vi "Singleton.vi"(8 "error in (no error)":errorcluster) -> (0 "error out":errorcluster, 1 "RequestQueue":refnum<queue>, 3 "MDPtrMgrDVR":refnum<data-value>)   [LabVIEW 2017, in "MDPtr.lvlib" / "MDPtrMgr.lvclass"]
uses:
  MDPtrMgr.lvclass
  Factory/Def-Request.ctl
  Factory/Def-Respone.ctl
  MDPtr TypeDef/MDPtr DataFrame-Memory.ctl
  MDPtr TypeDef/MDPtr DataFrame-Common.ctl
  <vilib>/Utility/Data Type/Type Definitions/Data Type.ctl
  Factory/Def-MDPtrQ.ctl
  <vilib>/Utility/Data Type/NI_Data Type.lvlib
  MDPtr.lvlib
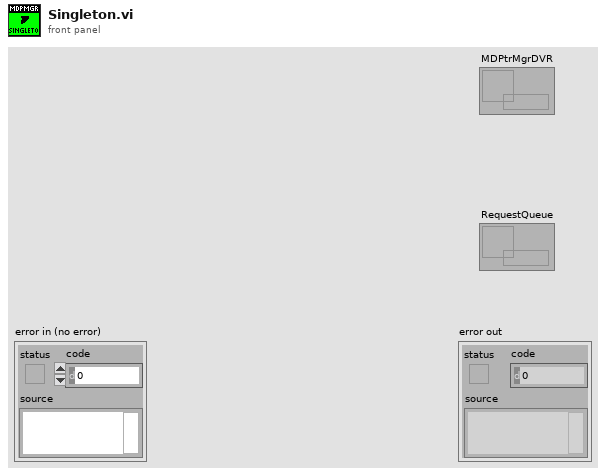
[diagram p1: front panel]
types:
  T1 = typedef "MDPtr.lvlib/MDPtrMgr.lvclass/Def-Request.ctl" = cluster{"Type":enum16{"DVR", "Queue"}, "Cache Length":i32, "ResponeQueue":refnum<queue>}
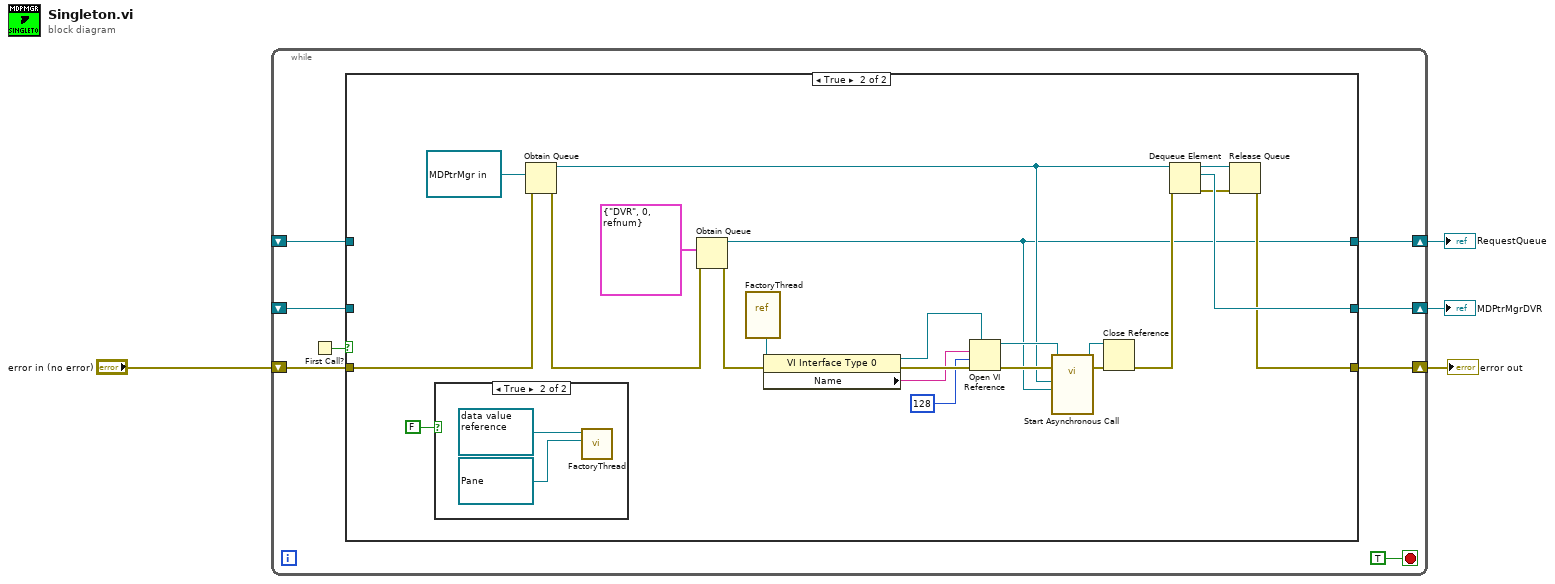
[diagram p0: block diagram]
diagram:
  n1 = while {
    shift-right: [w10] -> w2
    shift-left: "error in (no error)" -> [w12]
    shift-right: [w11] -> w3
    shift-left: _ -> [w7]
    shift-right: [w6] -> w1
    shift-left: _ -> [w5]
    stop <- TRUE stop-if-true
    n2 = First Call?() -> (First Call?: T/F=w8:bool)
    n3 = case shown="True" w8 {
      tunnel: w12 -> [w14 w37]
      tunnel: [w15 w27] -> w11
      tunnel: [w14 w23] -> w10
      tunnel: w7 -> [w15 _]
      tunnel: [w13 w18] -> w6
      tunnel: w5 -> [w13 _]
      frame False {
      }
      frame True {
        n4 = case shown="True" FALSE {
          frame False {
          }
          frame True {
            n5 = call "FactoryThread.vi"("SyncUpQueue"=refnum<queue> refnum ("queue out"), "ReturnQUEUE"=refnum<queue> refnum ("queue out")) -> ()  [unwired: 10 in]
          }
        }
        n6 = Obtain Queue(element data type=refnum<data-value> refnum ("data value reference"), error in (no error)=w37) -> (queue out=w29:refnum<queue>, error out=w20:errorcluster)  [unwired: 3 in, 1 out]
        n7 = Obtain Queue(element data type=T1 {"Type"=enum."DVR", "Cache Length"=0, "ResponeQueue"=refnum}, error in (no error)=w20) -> (queue out=w18:refnum<queue>, error out=w19:errorcluster)  [unwired: 3 in, 1 out]
        n8 = vi-ref "FactoryThread.vi"() -> (w34:refnum<vi>)
        n9 = property class="VI Interface Type 0"(reference=w34, error in=w19) -> (reference out=w16:refnum<vi>, error out=w35:errorcluster, "Name"=w33:string)
        n10 = Open VI Reference(type specifier VI Refnum (for type only)=w16, vi path=w33, options=128, error in (no error)=w35) -> (vi reference=w30:refnum<vi>, error out=w36:errorcluster)  [unwired: 2 in]
        n11 = call-by-ref "Start Asynchronous Call"(reference=w30, error in=w36, "SyncUpQueue"=w18, "ReturnQUEUE"=w29) -> (reference out=w28:refnum<vi>, error out=w31:errorcluster)  [unwired: 10 in]
        n12 = Close Reference(reference=w28, error in (no error)=w31) -> (error out=w26:errorcluster)
        n13 = Dequeue Element(queue=w29, error in (no error)=w26) -> (queue out=w22:refnum<queue>, element=w27:refnum<data-value>, error out=w25:errorcluster)  [unwired: 1 in, 1 out]
        n14 = Release Queue(queue=w22, error in (no error)=w25) -> (error out=w23:errorcluster)  [unwired: 1 in, 2 out]
      }
    }
  }
  "error out" <- w2
  "MDPtrMgrDVR" <- w3
  "RequestQueue" <- w1
